vi "Log Error.vi"(8 "error in (no error)":errorcluster, 11 "S4GUI in":refnum<class "S4GUI.lvclass">) -> (0 "error out":errorcluster, 3 "S4GUI out":refnum<class "S4GUI.lvclass">)   [LabVIEW 2018, in "S4GUI.lvclass"]
uses:
  S4GUI.lvclass
  S4GUI.lvclass/S4GUI.ctl
  Log/Log.lvclass
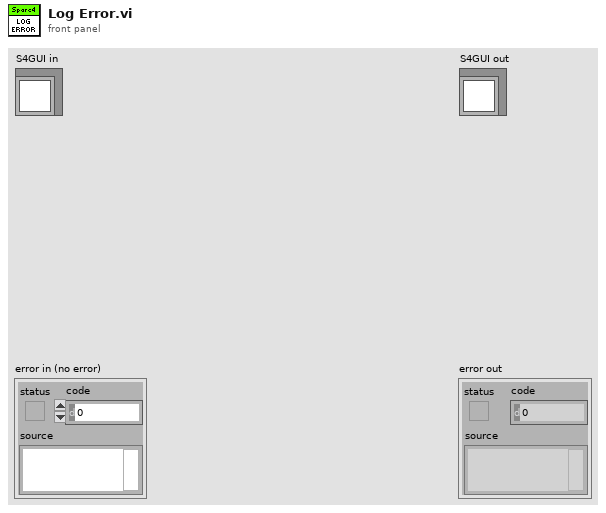
[diagram p1: front panel]
types:
  T1 = enum16{"INFO ", "TRACE", "DEBUG", "WARN ", "ERROR", "FATAL", "OTHER"}
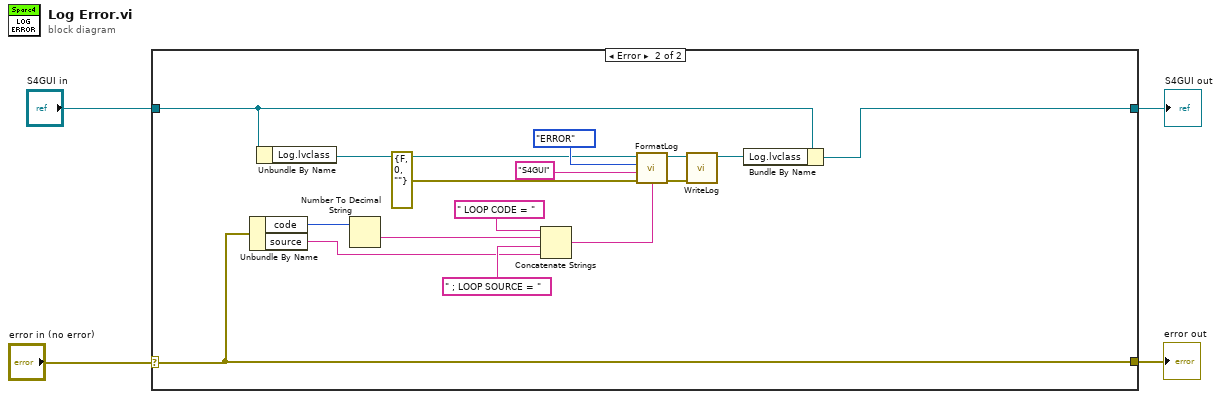
[diagram p0: block diagram]
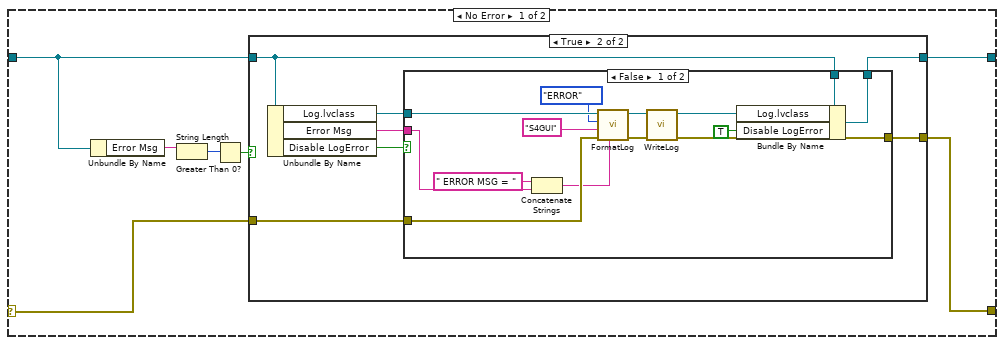
[diagram p2: hidden frame]
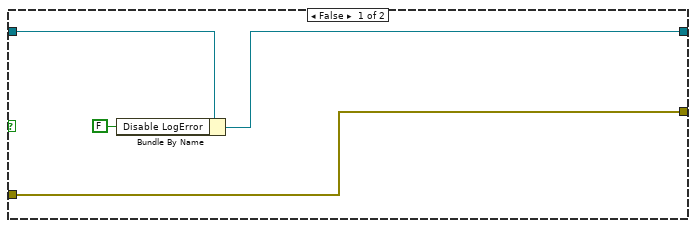
[diagram p3: hidden frame]
diagram:
  n1 = case shown="Error" "error in (no error)" {
    selector: "error in (no error)" -> [w6 w54]
    tunnel: [w5 w54] -> w3
    tunnel: [w7 w43] -> w1
    tunnel: "S4GUI in" -> [w8 w44]
    frame No Error {
      n2 = Unbundle By Name(w8) -> ("Error Msg"=w11:string)
      n3 = String Length(string=w11) -> (length=w10:i32)
      n4 = Greater Than 0?(x=w10) -> (x > 0?=w9:bool)
      n5 = case shown="True" w9 {
        tunnel: w8 -> [w15 w20]
        tunnel: [w14 w19] -> w7
        tunnel: w6 -> [w12 w17]
        tunnel: [w12 w16] -> w5
        frame False {
          n6 = Bundle By Name(cluster=w15, "Disable LogError"=FALSE) -> (w14:refnum<class "S4GUI.lvclass">)
        }
        frame True {
          n7 = Unbundle By Name(w20) -> ("Log.lvclass"=w21:refnum<class "Log.lvclass">, "Error Msg"=w22:string, "Disable LogError"=w18:bool)
          n8 = case shown="False" w18 {
            tunnel: w22 -> [w25 _]
            tunnel: w21 -> [w33 _]
            tunnel: w20 -> [w36 w38]
            tunnel: [w35 w38] -> w19
            tunnel: w17 -> [w29 w37]
            tunnel: [w28 w37] -> w16
            frame False {
              n9 = Concatenate Strings(" ERROR MSG = " ("string"), w25) -> (w24:string)
              n10 = call-dynamic "FormatLog.vi"("log input"=w24, "error in (no error)"=w29, "System"="S4GUI", "Type"=T1."ERROR", "Log in"=w33) -> ("error out"=w30:errorcluster, "Log out"=w32:refnum<class "Log.lvclass">)  [unwired: 5 in]
              n11 = call-dynamic "WriteLog.vi"("error in (no error)"=w30, "Log in"=w32) -> ("error out"=w28:errorcluster, "Log out"=w31:refnum<class "Log.lvclass">)  [unwired: 8 in]
              n12 = Bundle By Name(cluster=w36, "Log.lvclass"=w31, "Disable LogError"=TRUE) -> (w35:refnum<class "S4GUI.lvclass">)
            }
            frame True {
            }
          }
        }
      }
    }
    frame Error {
      n13 = Unbundle By Name(w54) -> ("code"=w42:i32, "source"=w39:string)
      n14 = Unbundle By Name(w44) -> ("Log.lvclass"=w46:refnum<class "Log.lvclass">)
      n15 = Number To Decimal String(number=w42) -> (decimal integer string=w41:string)  [unwired: 1 in]
      n16 = Concatenate Strings(" LOOP CODE = " ("string"), w41, " ; LOOP SOURCE = " ("string"), w39) -> (w48:string)
      n17 = call-dynamic "FormatLog.vi"("log input"=w48, "error in (no error)"=errorcluster {"status"=FALSE, "code"=0, "source"=""}, "System"="S4GUI", "Type"=T1."ERROR", "Log in"=w46) -> ("error out"=w51:errorcluster, "Log out"=w53:refnum<class "Log.lvclass">)  [unwired: 5 in]
      n18 = call-dynamic "WriteLog.vi"("error in (no error)"=w51, "Log in"=w53) -> ("Log out"=w52:refnum<class "Log.lvclass">)  [unwired: 8 in, 1 out]
      n19 = Bundle By Name(cluster=w44, "Log.lvclass"=w52) -> (w43:refnum<class "S4GUI.lvclass">)
    }
  }
  "error out" <- w3
  "S4GUI out" <- w1
